vi "Newmark-Clear.vi"(0 "Table VRN IN":refnum<visa-resource-name>="COM9", 2 "Bool Refnum":refnum<vi>, 11 "Error IN":errorcluster) -> (4 "Table VRN OUT":refnum<visa-resource-name>="COM9", 15 "Error OUT":errorcluster)   [LabVIEW 2011]
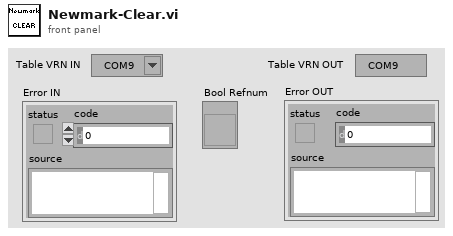
[diagram p1: front panel]
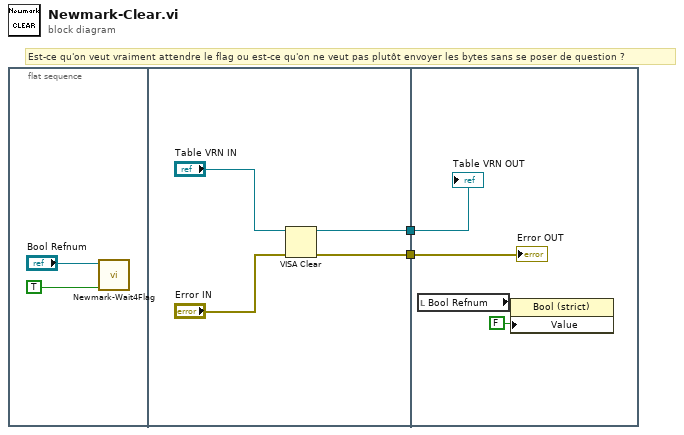
[diagram p0: block diagram]
diagram:
  # "Est-ce qu'on veut vraiment attendre le flag ou est-ce qu'on ne veut pas plutôt envoyer les bytes sans se poser de question ?"
  n1 = flat-sequence {
    tunnel: [w8] -> w2
    tunnel: [w7] -> w1
    tunnel: w2 -> [w12]
    tunnel: w1 -> [w11]
    frame #0 {
      n2 = call "Newmark-Wait4Flag.vi"("Raise Flag ?"=TRUE, "Ctl Refnum IN"="Bool Refnum") -> ()  [unwired: 8 in, 2 out]
    }
    frame #1 {
      n3 = VISA Clear(VISA resource name="Table VRN IN", error in (no error)="Error IN") -> (VISA resource name out=w8:refnum<visa-resource-name>, error out=w7:errorcluster)
    }
    frame #2 {
      n4 = local read "Bool Refnum"() -> (w10:refnum<vi>)
      n5 = property class="Bool (strict)"(reference=w10, "Value"=FALSE) -> ()  [unwired: 1 in, 2 out]
      "Error OUT" <- w11
      "Table VRN OUT" <- w12
    }
  }
